vi "move_.vi"(0 "Enum":enum16{"hold", "f", "b"}(ring), 2 "delay":u32, 3 "D":dbl) -> ()   [LabVIEW 2017]
uses:
  Untitled Project 6/GlobalVar.vi
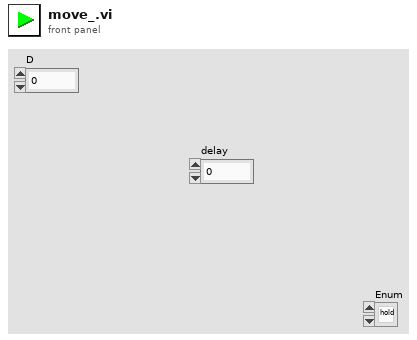
[diagram p1: front panel]
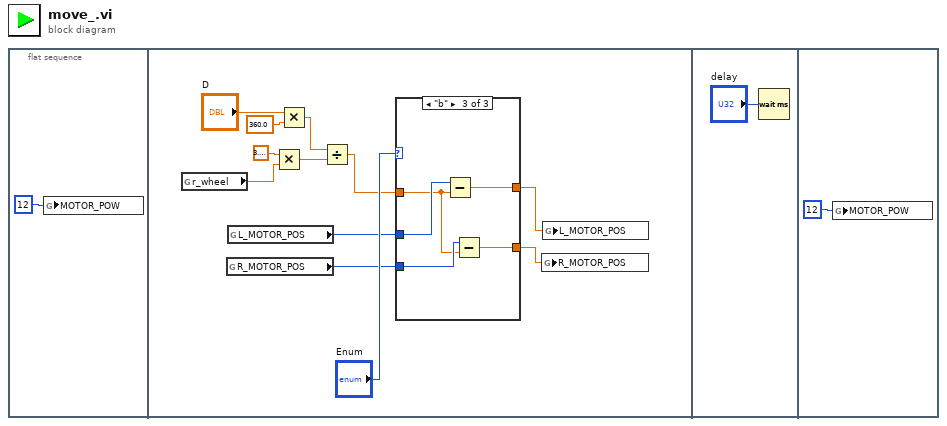
[diagram p0: block diagram]
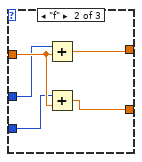
[diagram p3: hidden frame]
diagram:
  n1 = flat-sequence {
    frame #0 {
      n2 = global write "GlobalVar.vi" "MOTOR_POW"(i8 12 ("MOTOR_POW")) -> ()
    }
    frame #1 {
      n3 = global read "GlobalVar.vi" "r_wheel"() -> (w2:dbl)
      n4 = global read "GlobalVar.vi" "R_MOTOR_POS"() -> (w6:i32)
      n5 = global read "GlobalVar.vi" "L_MOTOR_POS"() -> (w7:i32)
      n6 = Multiply(x=3.141592653589793, y=w2) -> (x*y=w9:dbl)
      n7 = Multiply(x="D", y=360.0) -> (x*y=w10:dbl)
      n8 = Divide(x=w10, y=w9) -> (x/y=w5:dbl)
      n9 = case shown="\"b\"" "Enum" {
        tunnel: w7 -> [w15 w19 w25]
        tunnel: w6 -> [w14 w18 w24]
        tunnel: w5 -> [_ w20 w23]
        tunnel: [w15 w16 w22] -> w4
        tunnel: [w14 w17 w21] -> w3
        frame "hold", Default {
        }
        frame "f" {
          n10 = Add(x=w19, y=w20) -> (x+y=w16:dbl)
          n11 = Add(x=w18, y=w20) -> (x+y=w17:dbl)
        }
        frame "b" {
          n12 = Subtract(x=w25, y=w23) -> (x-y=w22:dbl)
          n13 = Subtract(x=w24, y=w23) -> (x-y=w21:dbl)
        }
      }
      n14 = global write "GlobalVar.vi" "R_MOTOR_POS"(w3) -> ()
      n15 = global write "GlobalVar.vi" "L_MOTOR_POS"(w4) -> ()
    }
    frame #2 {
      n16 = Wait (ms)(milliseconds to wait="delay") -> ()  [unwired: 1 out]
    }
    frame #3 {
      n17 = global write "GlobalVar.vi" "MOTOR_POW"(i8 12 ("MOTOR_POW")) -> ()
    }
  }
